vi "LakeShore Ramp Com.vi"(2 "command text in":string[](array[string]), 3 "option":T2) -> (1 "Command text out":string[][](array[string]))   [LabVIEW 2020]
uses:
  Ctl/option.ctl
  LSRamp.ctl
panel:
  in  "LSRamp":T1={"VISA Resource Name"="", "extra wait"=0, "start (K/W)"=1e-09, "end (K/W)"=0.001, "Sweep Time (H:M:S)"=3600.0, "Mapping"=FALSE, "Parameter"=FALSE, "Loop"=FALSE} {"Sweep Time (H:M:S)" format="%<%H:%M:%S>t"; "extra wait" min=0; "start (K/W)" format="%#.7e"; "end (K/W)" format="%#.7e"}
  in  "enter":bool
  in  "cancel":bool
  # "LakeShore Ramp"
  # "Log"
  # "Start Temp(K)/Power(W)"
  # "Sweep Time (HH:MM:SS)"
  # "End Temp(K)/Power(W)"
  # "Linear"
  # "seconds"
  # "AND wait extra"
  # "Power"
  # "Temp"
  # "VISA Name"
  # "Loop 2"
  # "Loop 1"
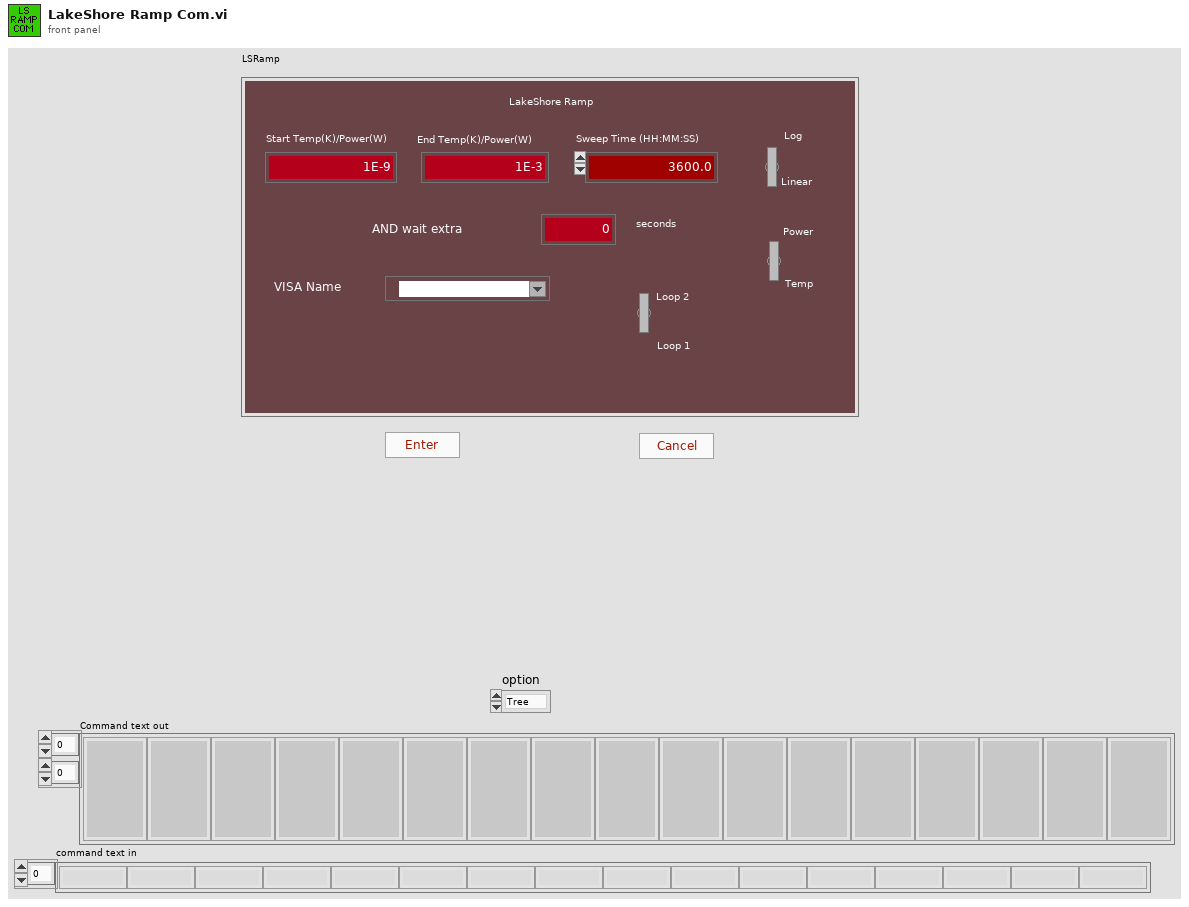
[diagram p1: front panel]
types:
  T1 = typedef "LSRamp.ctl" = cluster{"VISA Resource Name":refnum<visa-resource-name>, "extra wait":i32, "start (K/W)":dbl, "end (K/W)":dbl, "Sweep Time (H:M:S)":dbl, "Mapping":bool, "Parameter":bool, "Loop":bool}
  T2 = typedef "option.ctl" = enum16{"Tree", "List"}
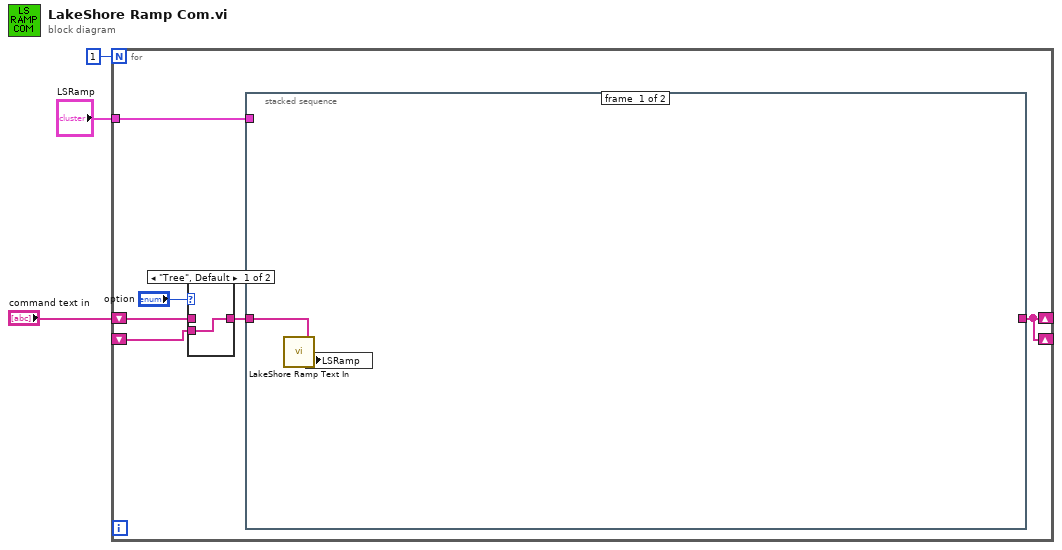
[diagram p0: block diagram]
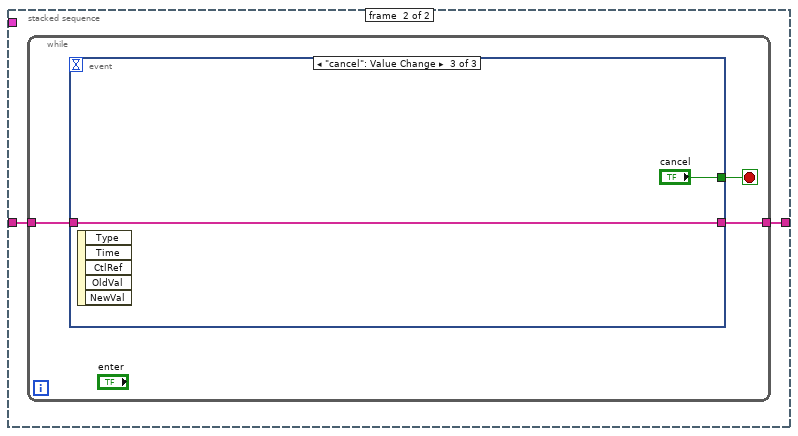
[diagram p3: hidden frame]
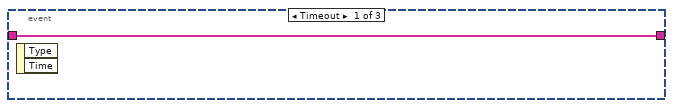
[diagram p4: hidden frame]
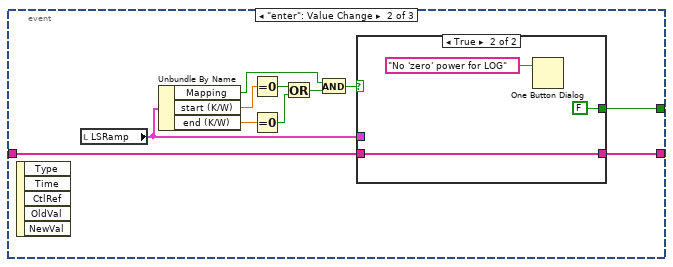
[diagram p5: hidden frame]
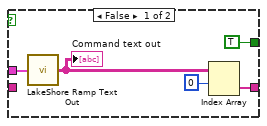
[diagram p6: hidden frame]
diagram:
  n1 = for {
    N: 1 -> [_]
    shift-right: [w6] -> _
    shift-left: _ -> [w8]
    shift-right: [w6] -> _
    shift-left: "command text in" -> [w7]
    tunnel: "LSRamp" -> [w4]
    n2 = case shown="\"Tree\", Default" "option" {
      tunnel: [w10 w11] -> w9
      tunnel: w8 -> [w10 _]
      tunnel: w7 -> [_ w11]
      frame "Tree", Default {
      }
      frame "List" {
      }
    }
    n3 = stacked-sequence {
      tunnel: [_ w15] -> w6
      tunnel: w9 -> [w13 w14]
      tunnel: w4 -> [_ _]
      frame #0 {
        n4 = call "LakeShore Ramp Text In.vi"("command text in"=w13) -> ("LSRamp"=w12:T1)  [unwired: 4 in]
        n5 = local write "LSRamp"(w12) -> ()
      }
      frame #1 {
        n6 = while {
          tunnel: [w17] -> w15
          tunnel: w14 -> [w16]
          stop <- w18 stop-if-true
          n7 = event shown="[2] \"cancel\": Value Change" {
            selector: _ -> [_ _ _]
            dyn-events: _ -> [_ _ _]
            timeout: _ -> [_ _ _]
            tunnel: [_ w20 "cancel"] -> w18
            tunnel: [w19 w30 w39] -> w17
            tunnel: w16 -> [w19 w21 w39]
            event Timeout {
              n8 = event-data() -> ()  [unwired: 1 in, 2 out]
            }
            event "enter": Value Change {
              n9 = event-data() -> ()  [unwired: 1 in, 5 out]
              n10 = local read "LSRamp"() -> (w29:T1)
              n11 = Unbundle By Name(w29) -> ("Mapping"=w24:bool, "start (K/W)"=w27:dbl, "end (K/W)"=w26:dbl)
              n12 = Equal To 0?(x=w27) -> (x = 0?=w28:bool)
              n13 = Equal To 0?(x=w26) -> (x = 0?=w25:bool)
              n14 = Or(x=w28, y=w25) -> (x .or. y?=w23:bool)
              n15 = And(x=w24, y=w23) -> (x .and. y?=w22:bool)
              n16 = case shown="True" w22 {
                tunnel: [w34 w38] -> w30
                tunnel: w29 -> [w32 _]
                tunnel: w21 -> [_ w38]
                tunnel: [TRUE FALSE] -> w20
                frame False {
                  n17 = call "LakeShore Ramp Text Out.vi"("LSRamp"=w32) -> ("Command text"=w31:string[][])
                  "Command text out" <- w31
                  n18 = Index Array(array=w31, index (row)=0) -> (element=w34:string[])  [unwired: 1 in]
                }
                frame True {
                  n19 = One Button Dialog(message="No 'zero' power for LOG") -> ()  [unwired: 1 in, 1 out]
                }
              }
            }
            event "cancel": Value Change {
              n20 = event-data() -> ()  [unwired: 1 in, 5 out]
            }
          }
        }
      }
    }
  }
